vi "start.vi"(8 "error in (no error)":errorcluster, 11 "HSDIO in":refnum<class "HSDIO.lvclass">) -> (0 "error out":errorcluster, 3 "HSDIO out":refnum<class "HSDIO.lvclass">)   [LabVIEW 2013, in "HSDIO.lvclass"]
uses:
  HSDIO.lvclass
  HSDIO_settings.ctl
  <instrlib>/niHSDIO/niHSDIO.llb/niHSDIO_ctl Trigger Script - trigID Values (Ring).ctl
  <instrlib>/niHSDIO/niHSDIO.llb/niHSDIO_ctl Trigger Source Values (Ring).ctl
  <instrlib>/niHSDIO/niHSDIO.llb/niHSDIO_ctl Trigger DigEdge - Edge Values (Ring).ctl
  <instrlib>/niHSDIO/niHSDIO.llb/niHSDIO_ctl Trigger DigLvl - Level Values (Ring).ctl
  waveform.ctl
  HSDIO.lvclass/HSDIO.ctl
  Experiment/Globals.vi
panel:
  out "HSDIO Settings":T1={"Enable HSDIO Pulses"=FALSE, "Resource Name"="PXI1Slot6", "Clock Rate"=20000000.0, "Array of Script Triggers"=[], "Pulse Generation Script"="script script1\n     Generate RedTrap_compress_temp\nend script", "Start Trigger"={"Wait for start trigger?"=FALSE, "source (PFI 0)"="PFI0", "edge (rising)"=12, "description"=""}, "Hardware alignment quantum\n(in samples)"=1, "Inital State"="", "Idle State"="", "Active Channels"="", "Array of Waveforms"=[], "description"=""} {"Hardware alignment quantum\n(in samples)" min=1 step=1; "Array of Script Triggers"."level" items=["High Level"=34, "Low Level"=35]; "Array of Script Triggers"."edge" items=["Rising Edge"=12, "Falling Edge"=13]; "Start Trigger"."edge (rising)" items=["Rising Edge"=12, "Falling Edge"=13]; "Clock Rate" min=0.0 max=200000000.0 format="%.2p"}
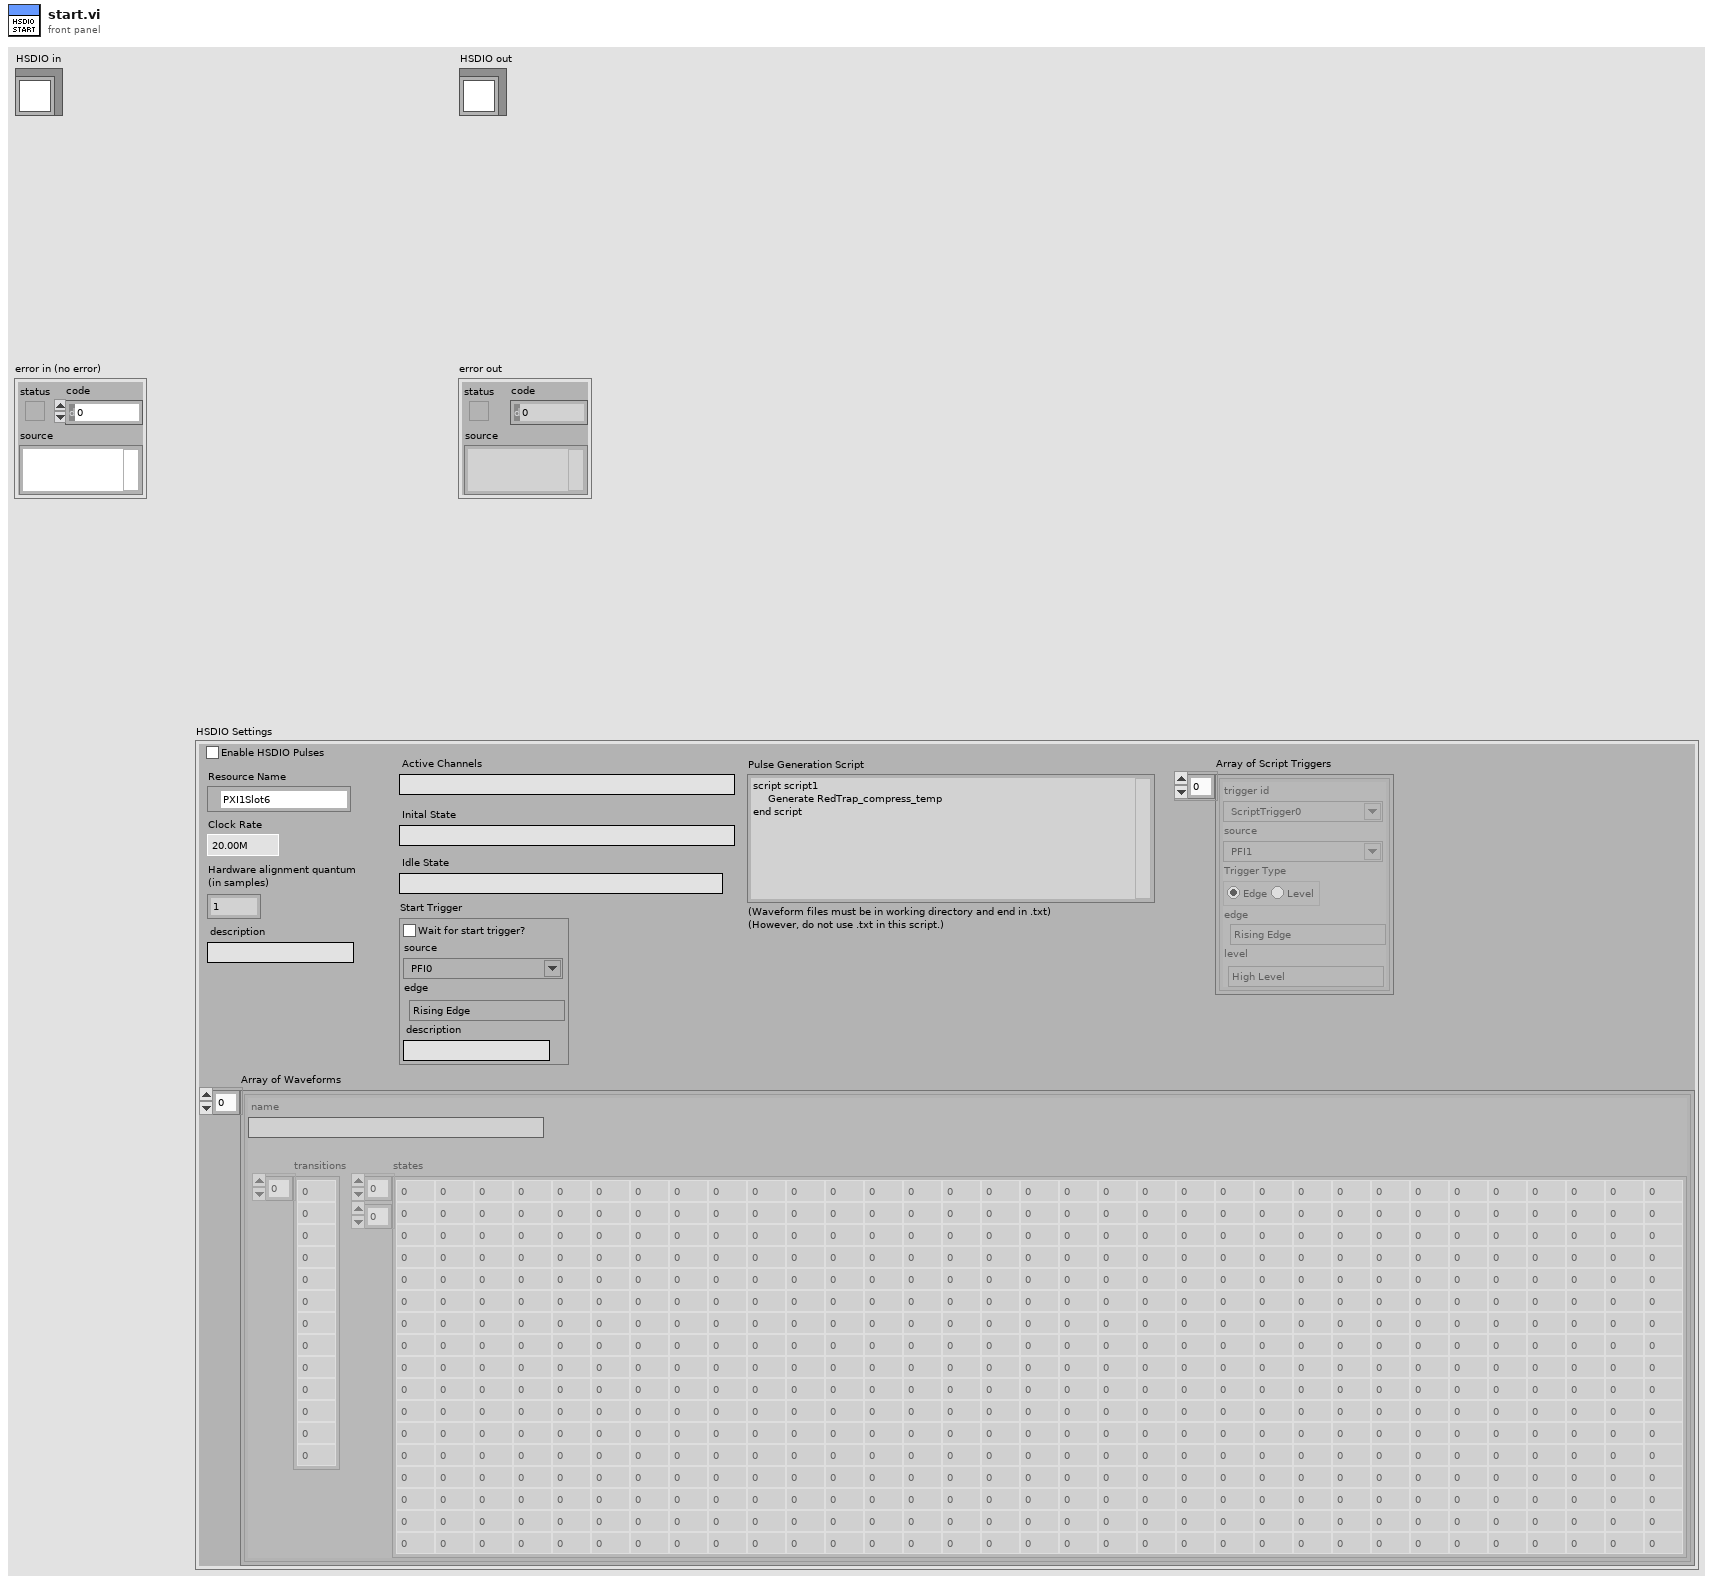
[diagram p1: front panel]
types:
  T1 = typedef "HSDIO.lvclass/HSDIO_settings.ctl" = cluster{"Enable HSDIO Pulses":bool, "Resource Name":refnum<k15>, "Clock Rate":dbl, "Array of Script Triggers":cluster{"trigger id (script trigger 0)":T2, "source (PFI 0)":T3, "Trigger Type":enum32{"Edge", "Level"}, "edge":T4, "level":T5}[], "Pulse Generation Script":string, "Start Trigger":cluster{"Wait for start trigger?":bool, "source (PFI 0)":T3, "edge (rising)":T4, "description":string}, "Hardware alignment quantum\n(in samples)":u16, "Inital State":string, "Idle State":string, "Active Channels":string, "Array of Waveforms":T6[], "description":string}
  T2 = typedef "niHSDIO_ctl Trigger Script - trigID Values (Ring).ctl" = string
  T3 = typedef "niHSDIO_ctl Trigger Source Values (Ring).ctl" = string
  T4 = typedef "niHSDIO_ctl Trigger DigEdge - Edge Values (Ring).ctl" = i32
  T5 = typedef "niHSDIO_ctl Trigger DigLvl - Level Values (Ring).ctl" = i32
  T6 = typedef "HSDIO.lvclass/waveform.ctl" = cluster{"name":string, "transitions":u32[], "states":u8[][]}
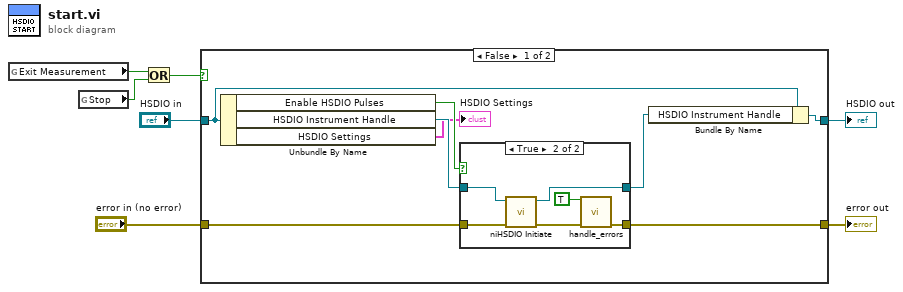
[diagram p0: block diagram]
diagram:
  n1 = global read "Globals.vi" "Exit Measurement"() -> (w3:bool)
  n2 = global read "Globals.vi" "Stop"() -> (w4:bool)
  n3 = Or(x=w3, y=w4) -> (x .or. y?=w2:bool)
  n4 = case shown="False" w2 {
    tunnel: [w9 w24] -> w5
    tunnel: [w11 w25] -> w6
    tunnel: "HSDIO in" -> [w12 w25]
    tunnel: "error in (no error)" -> [w8 w24]
    frame False {
      n5 = Unbundle By Name(w12) -> ("Enable HSDIO Pulses"=w15:bool, "HSDIO Instrument Handle"=w14:refnum<k15>, "HSDIO Settings"=→"HSDIO Settings":T1)
      n6 = case shown="True" w15 {
        tunnel: w8 -> [w17 w23]
        tunnel: [w17 w19] -> w9
        tunnel: w14 -> [w16 w22]
        tunnel: [w16 w21] -> w13
        frame False {
        }
        frame True {
          n7 = call <instrlib>:"niHSDIO Initiate.vi"("error in (no error)"=w23, "instrument handle"=w22) -> ("error out"=w18:errorcluster, "instrument handle out"=w21:refnum<k15>)  [unwired: 8 in]
          n8 = call "handle_errors.vi"("Exit Operation"=TRUE ("Exit Measurement"), "error in (no error)"=w18) -> ("error out"=w19:errorcluster)  [unwired: 13 in]
        }
      }
      n9 = Bundle By Name(cluster=w12, "HSDIO Instrument Handle"=w13) -> (w11:refnum<class "HSDIO.lvclass">)
    }
    frame True {
    }
  }
  "error out" <- w5
  "HSDIO out" <- w6
